vi "Open GUI.vi"(8 "error in (no error)":errorcluster, 11 "PluginGUI in":refnum<class "PluginGUI.lvclass">) -> (0 "error out":errorcluster, 3 "PluginGUI out":refnum<class "PluginGUI.lvclass">)   [LabVIEW 2020, in "VolatusGUI.lvlib" / "PluginGUI.lvclass"]
uses:
  PluginGUI.lvclass
  PluginGUI.lvclass/PluginGUI.ctl
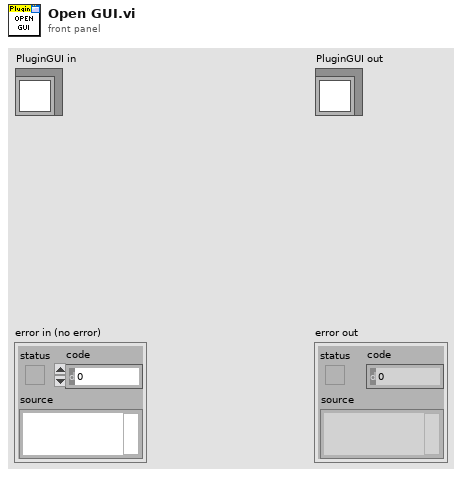
[diagram p1: front panel]
types:
  T1 = enum32{"Invalid", "Standard", "Closed", "Hidden", "Minimized", "Maximized"}
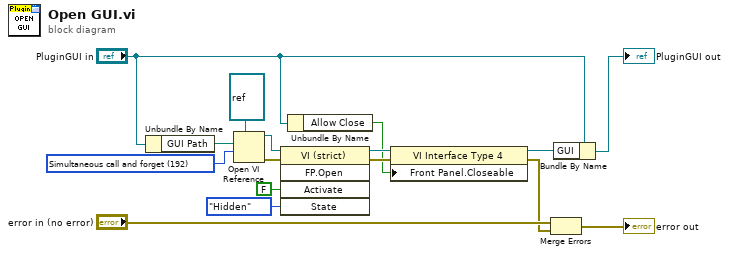
[diagram p0: block diagram]
diagram:
  w14 = 192 items=["Record modifications"=1, "Open templates for editing"=2, "Prompt user to save"=4, "Prepare for reentrant run"=8, "Prompt to find missing subVIs"=16, "Hide loading dialog box"=32, "Enable simultaneous calls"=64, "Prepare to call and forget"=128, "Simultaneous call and forget"=192, "Prepare to call and collect"=256, "Simultaneous call and collect"=320]
  n1 = Unbundle By Name("PluginGUI in") -> ("GUI Path"=w15:path)
  n2 = Open VI Reference(type specifier VI Refnum (for type only)=refnum<vi> refnum, vi path=w15, options=w14) -> (vi reference=w9:refnum<vi>, error out=w10:errorcluster)  [unwired: 3 in]
  n3 = invoke class="VI (strict)" method="FP.Open"(reference=w9, error in=w10, "Activate"=FALSE ("Activate?"), "State"=T1."Hidden") -> (reference out=w6:refnum<vi>, error out=w5:errorcluster)  [unwired: 1 in, 3 out]
  n4 = Unbundle By Name("PluginGUI in") -> ("Allow Close"=w3:bool)
  n5 = property class="VI Interface Type 4"(reference=w6, error in=w5, "Front Panel.Closeable"=w3) -> (reference out=w2:refnum<vi>, error out=w1:errorcluster)
  n6 = Merge Errors("error in (no error)", w1) -> (→"error out":errorcluster)
  n7 = Bundle By Name(cluster="PluginGUI in", "GUI"=w2) -> (→"PluginGUI out":refnum<class "PluginGUI.lvclass">)
